vi "GeradorDegrau.vi"(9 "IA State Input":T1={"our_robots"=[], "enemy_robots"=[], "balls"=[], "geometry"={"line_width"=0, "field_length"=0, "field_width"=0, "boundary_width"=0, "referee_width"=0, "goal_width"=0, "goal_depth"=0, "goal_wall_width"=0, "center_circle_radius"=0, "defense_radius"=0, "defense_stretch"=0, "free_kick_from_defense_dist"=0, "penalty_spot_from_field_line_dist"=0, "penalty_line_from_spot_dist"=0}, "IA Judge"={"stage"="", "command"="", "our_goalie_id"=0.0, "enemy_goalie_id"=0.0, "command enum"=enum."Halt", "Time"=enum."Azul"}, "Received Timestamp"=timestamp(0 s since 1904-01-01), "Events"={"Touch"=FALSE, "Ball out"=FALSE, "id touch"=0.0, "Ball out of \nVision"=FALSE, "Ball inside \nGoalie area"=FALSE, "Robot not responding"=FALSE, "Robots responding status"=[1.0, 1.0, 1.0, 1.0, 1.0, 1.0], "Enemy Ball \nPossession"=FALSE, "Pass State"=FALSE, "id end of pass"=0.0, "Kick"=FALSE, "Id ini Possession"=0.0, "Ball Possesion"=FALSE, "Id Possesion"=0.0, "Direct Kick"=FALSE}}, 10 "Robô":i32, 11 "Liga/Desliga":bool) -> ()   [LabVIEW 2018]
uses:
  Core/AI Input.ctl
  Core/AI Robot.ctl
  Intel/Functions Enum.ctl
  Intel/AttackerStates.ctl
  Path Planning/RRT/PathDests.ctl
  Path Planning/RRT/PathDest.ctl
  Core/AI Ball.ctl
  Core/Field Size.ctl
  Core/AI Judge.ctl
  Intel/Command Enum.ctl
  Util/Events/Events.ctl
panel:
  out "error out":errorcluster
  out "output waveform":waveform(dbl)
  in  "File path":path=path "C:/Users/lucas/Documents/RoboIME/GeradorDegrau/Degrau/dados.txt"
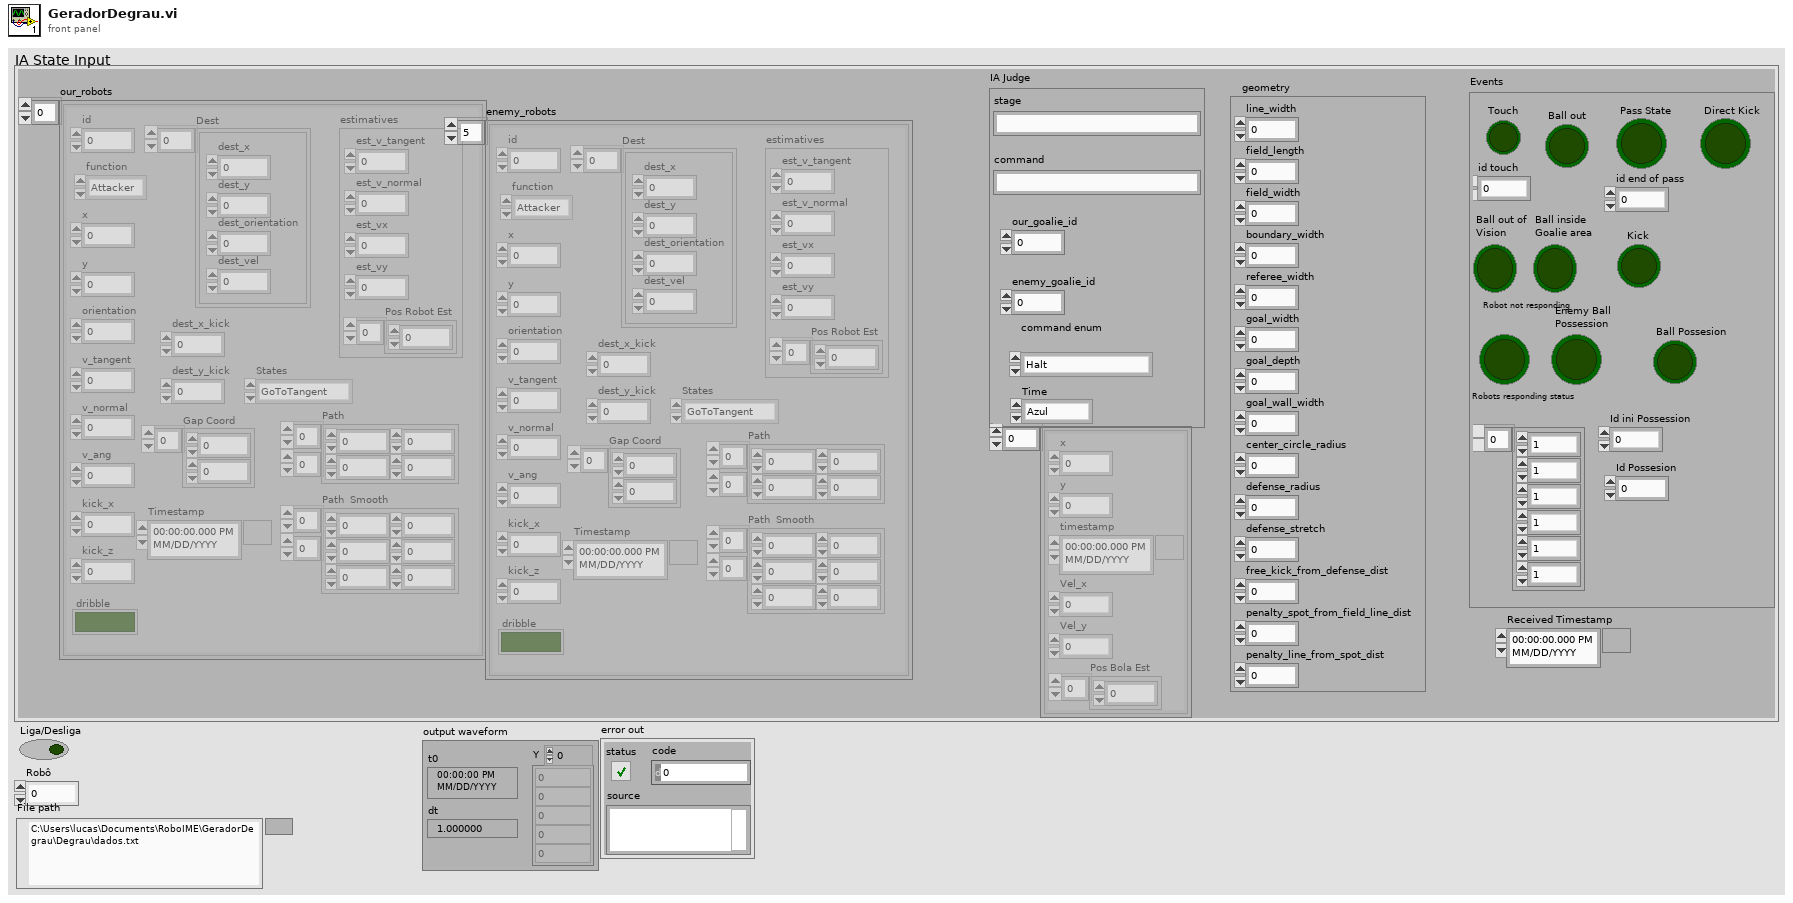
[diagram p1: front panel]
types:
  T1 = typedef "AI Input.ctl" = cluster{"our_robots":T2[], "enemy_robots":T2[], "balls":T7[], "geometry":T8, "IA Judge":T9, "Received Timestamp":timestamp, "Events":T11}
  T2 = typedef "AI Robot.ctl" = cluster{"id":u32, "function":T3, "x":dbl, "y":dbl, "orientation":dbl, "v_tangent":dbl, "v_normal":dbl, "v_ang":dbl, "kick_x":dbl, "kick_z":dbl, "dribble":bool, "Timestamp":timestamp, "estimatives":cluster{"est_v_tangent":dbl, "est_v_normal":dbl, "est_vx":dbl, "est_vy":dbl, "Pos Robot Est":dbl[]}, "dest_x_kick":dbl, "dest_y_kick":dbl, "Gap Coord":dbl[], "States":T4, "Path ":dbl[][], "Path  Smooth":dbl[][], "Dest":T5}
  T3 = typedef "Functions Enum.ctl" = enum16{"Attacker", "Goalie", "Defender", "Striker", "Goto 0", "Dummy", "Kicker", "ZigZag 0", "ZigZag 1", "ZigZag 2", "ZigZag 3", "ZigZag 4", "ZigZag 5", "ZigZag 6", "ZigZag 7", "ZigZag 8", ""}
  T4 = typedef "AttackerStates.ctl" = enum16{"Pass", "GoToTangent", "BallGetting", "GoToKick", ""}
  T5 = typedef "PathDests.ctl" = T6[]
  T6 = typedef "PathDest.ctl" = cluster{"dest_x":dbl, "dest_y":dbl, "dest_orientation":dbl, "dest_vel":dbl}
  T7 = typedef "AI Ball.ctl" = cluster{"x":dbl, "y":dbl, "timestamp":timestamp, "Vel_x":dbl, "Vel_y":dbl, "Pos Bola Est":dbl[]}
  T8 = typedef "Field Size.ctl" = cluster{"line_width":u32, "field_length":u32, "field_width":u32, "boundary_width":u32, "referee_width":u32, "goal_width":u32, "goal_depth":u32, "goal_wall_width":u32, "center_circle_radius":u32, "defense_radius":u32, "defense_stretch":u32, "free_kick_from_defense_dist":u32, "penalty_spot_from_field_line_dist":u32, "penalty_line_from_spot_dist":u32}
  T9 = typedef "AI Judge.ctl" = cluster{"stage":string, "command":string, "our_goalie_id":dbl, "enemy_goalie_id":dbl, "command enum":T10, "Time":enum16{"Azul", "Amarelo"}}
  T10 = typedef "Command Enum.ctl" = enum16{"Halt", "Stop", "Force Start", "PKA Normal Start", "Prepare Kickoff Ally", "PKE Normal Start", "Prepare Kickoff Enemy", "Prepare Penalty Ally", "PPA Normal Start", "Prepare Penalty Enemy", "PPE Normal Start", "Direct Free Enemy", "Direct Free Ally", "Indirect Free Enemy", "Indirect Free Ally", "Timeout Enemy", "Timeout Ally", "Goal Enemy", "Goal Ally", "Ball Placement Enemy", "Ball Placement Ally", "Normal Half Time", "Extra Time Break", "Extra Half Time", "None", "Post Game"}
  T11 = typedef "Events.ctl" = cluster{"Touch":bool, "Ball out":bool, "id touch":dbl, "Ball out of \nVision":bool, "Ball inside \nGoalie area":bool, "Robot not responding":bool, "Robots responding status":dbl[], "Enemy Ball \nPossession":bool, "Pass State":bool, "id end of pass":dbl, "Kick":bool, "Id ini Possession":dbl, "Ball Possesion":bool, "Id Possesion":dbl, "Direct Kick":bool}
  T12 = enum16{"open", "open or create", "create or replace", "create", "open (read only)"}
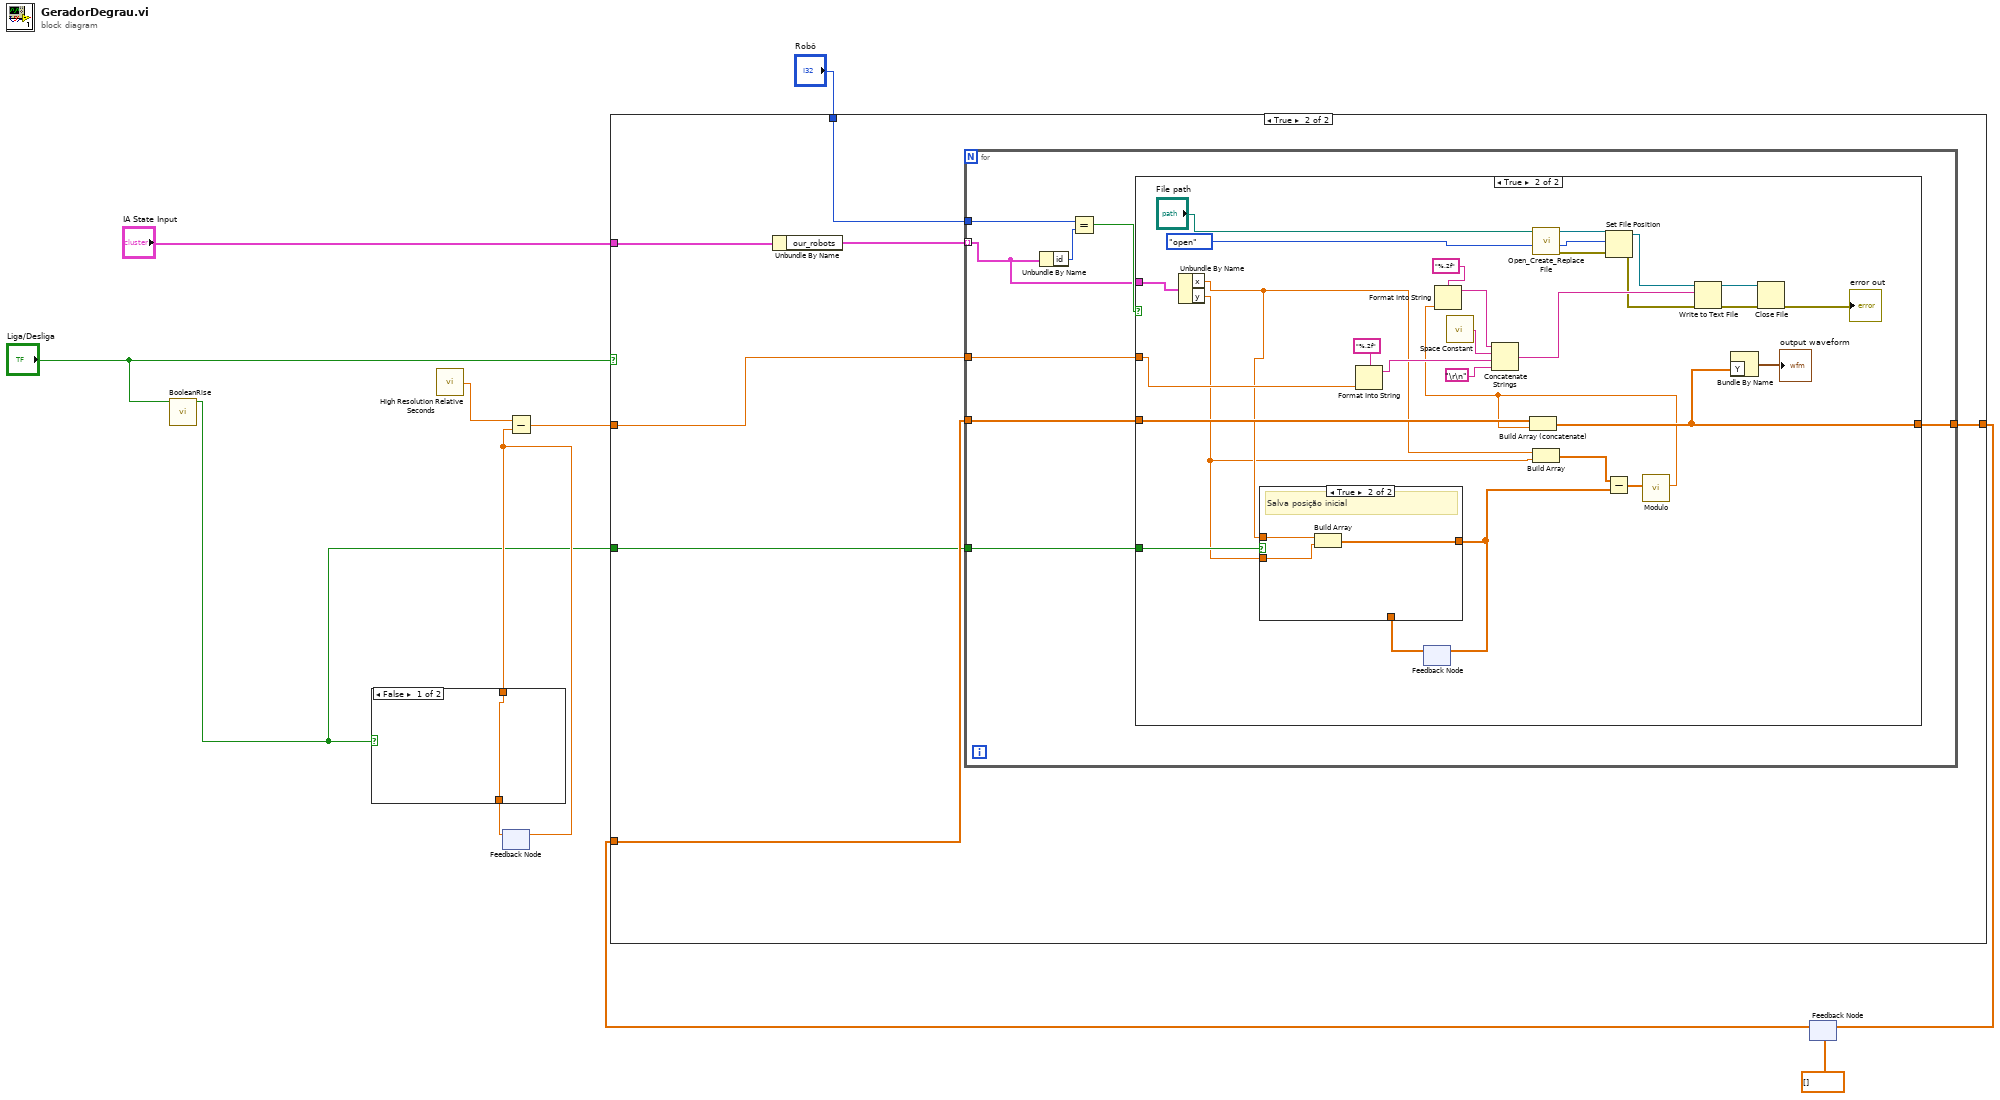
[diagram p0: block diagram]
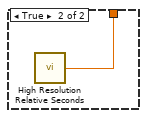
[diagram p2: hidden frame]
diagram:
  n1 = call "BooleanRise.vi"("Test Mode On"="Liga/Desliga") -> ("Boolean"=w1:bool)  [unwired: 10 in]
  n2 = call <vilib>:"High Resolution Relative Seconds.vi"() -> ("relative seconds"=w2:dbl)
  n3 = feedback #1() -> (w3:dbl)  [unwired: 1 in]
  n4 = case shown="False" w1 {
    tunnel: [w12 w13] -> w4
    tunnel: w3 -> [w12 _]
    frame False {
    }
    frame True {
      n5 = call <vilib>:"High Resolution Relative Seconds.vi"() -> ("relative seconds"=w13:dbl)
    }
  }
  n6 = feedback-in #1(w4) -> ()
  n7 = Subtract(x=w2, y=w4) -> (x-y=w5:dbl)
  n8 = feedback #2(dbl[] []) -> (w6:dbl[])
  n9 = case shown="True" "Liga/Desliga" {
    tunnel: "IA State Input" -> [_ w21]
    tunnel: "Robô" -> [_ w19]
    tunnel: [w14 w18] -> w8
    tunnel: w6 -> [w14 w17]
    tunnel: w5 -> [_ w16]
    tunnel: w1 -> [_ w15]
    frame False {
    }
    frame True {
      n10 = Unbundle By Name(w21) -> ("our_robots"=w20:T2[])
      n11 = for {
        tunnel: w20 -> [w26] mode=indexing
        tunnel: w19 -> [w28]
        tunnel: [w25] -> w18
        tunnel: w17 -> [w24]
        tunnel: w16 -> [w23]
        tunnel: w15 -> [w22]
        n12 = Unbundle By Name(w26) -> ("id"=w29:u32)
        n13 = Equal?(x=w28, y=w29) -> (x = y?=w27:bool)
        n14 = case shown="True" w27 {
          tunnel: w26 -> [_ w60]
          tunnel: [w30 w57] -> w25
          tunnel: w24 -> [w30 w58]
          tunnel: w23 -> [_ w42]
          tunnel: w22 -> [_ w38]
          frame False {
          }
          frame True {
            n15 = Unbundle By Name(w60) -> ("x"=w36:dbl, "y"=w35:dbl)
            n16 = Format Into String(format string="%.2f", w42) -> (resulting string=w41:string)  [unwired: 2 in, 1 out]
            n17 = feedback #3() -> (w37:dbl[])  [unwired: 1 in]
            n18 = case shown="True" w38 {
              tunnel: w36 -> [_ w64]
              tunnel: w35 -> [_ w63]
              tunnel: [w61 w62] -> w33
              tunnel: w37 -> [w61 _]
              frame False {
              }
              frame True {
                # "Salva posição inicial"
                n19 = Build Array(w64, w63) -> (w62:dbl[])
              }
            }
            n20 = feedback-in #3(w33) -> ()
            n21 = call <vilib>:"Space Constant.vi"() -> ("String"=w59:string)
            n22 = call <vilib>:"Open_Create_Replace File.vi"("function (open:0)"=T12."open", "file path"="File path") -> ("error out"=w47:errorcluster, "file size (bytes)"=w50:i32, "refnum"=w49:refnum<file>)  [unwired: 6 in, 1 out]
            n23 = Build Array(w36, w35) -> (w34:dbl[])
            n24 = Subtract(x=w34, y=w33) -> (x-y=w32:dbl[])
            n25 = Set File Position(offset (in bytes) (0)=w50, refnum=w49, error in=w47) -> (refnum out=w48:refnum<file>, error out=w46:errorcluster)  [unwired: 1 in]
            n26 = call "Modulo.vi"("2D vector"=w32) -> ("Modulo"=w31:dbl)  [unwired: 10 in]
            n27 = Format Into String(format string="%.2f", w31) -> (resulting string=w39:string)  [unwired: 2 in, 1 out]
            n28 = Concatenate Strings(w39, w59, w41, "\r\n") -> (w55:string)
            n29 = Build Array (concatenate)(w58, w31) -> (w57:dbl[])
            n30 = Write to Text File(file (use dialog)=w48, text=w55, error in=w46) -> (refnum out=w54:refnum<file>, error out=w45:errorcluster)  [unwired: 1 in, 1 out]
            n31 = Bundle By Name("Y"=w57) -> (→"output waveform":waveform(dbl))  [unwired: 1 in]
            n32 = Close File(refnum=w54, error in=w45) -> (error out=→"error out":errorcluster)  [unwired: 1 out]
          }
        }
      }
    }
  }
  n33 = feedback-in #2(w8) -> ()
